vi "Tran to CRC.vi"(5 "CheckSum？":bool, 7 "Count":bool, 8 "MessageFrame":refnum<k21>="ESP_1\nLRA110", 9 "校验算法名称":string="Anti_Add", 11 "CAN_commd":dbl[](array[numeric])=[50.0, 1.0, 11.0, 0.0, 0.0, 0.0, 0.0, 0.0, 0.0] caption="data") -> (1 "Output CAN Command":u8[](array[numeric]) format="%x", 2 "校验值":u64 format="%.0x", 3 "SignalsArryOut":dbl[](array[numeric]))   [LabVIEW 2020]
panel:
  out "CAN_Command_U8":u8[](array[numeric]) format="%.0x"
  # "speedStatus"
  # "counter"
  # "speed"
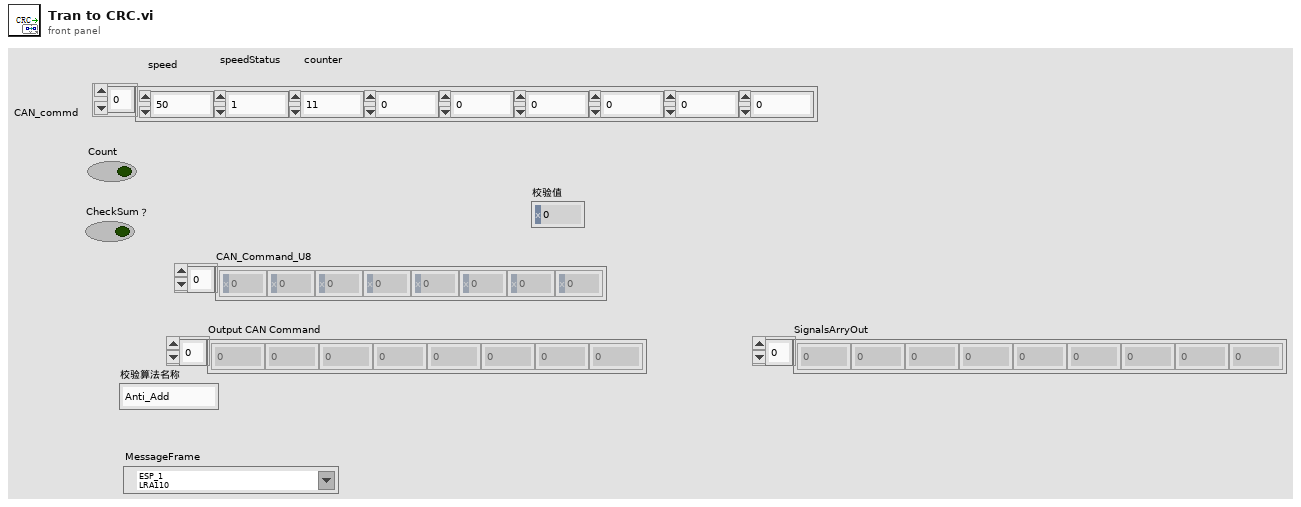
[diagram p1: front panel]
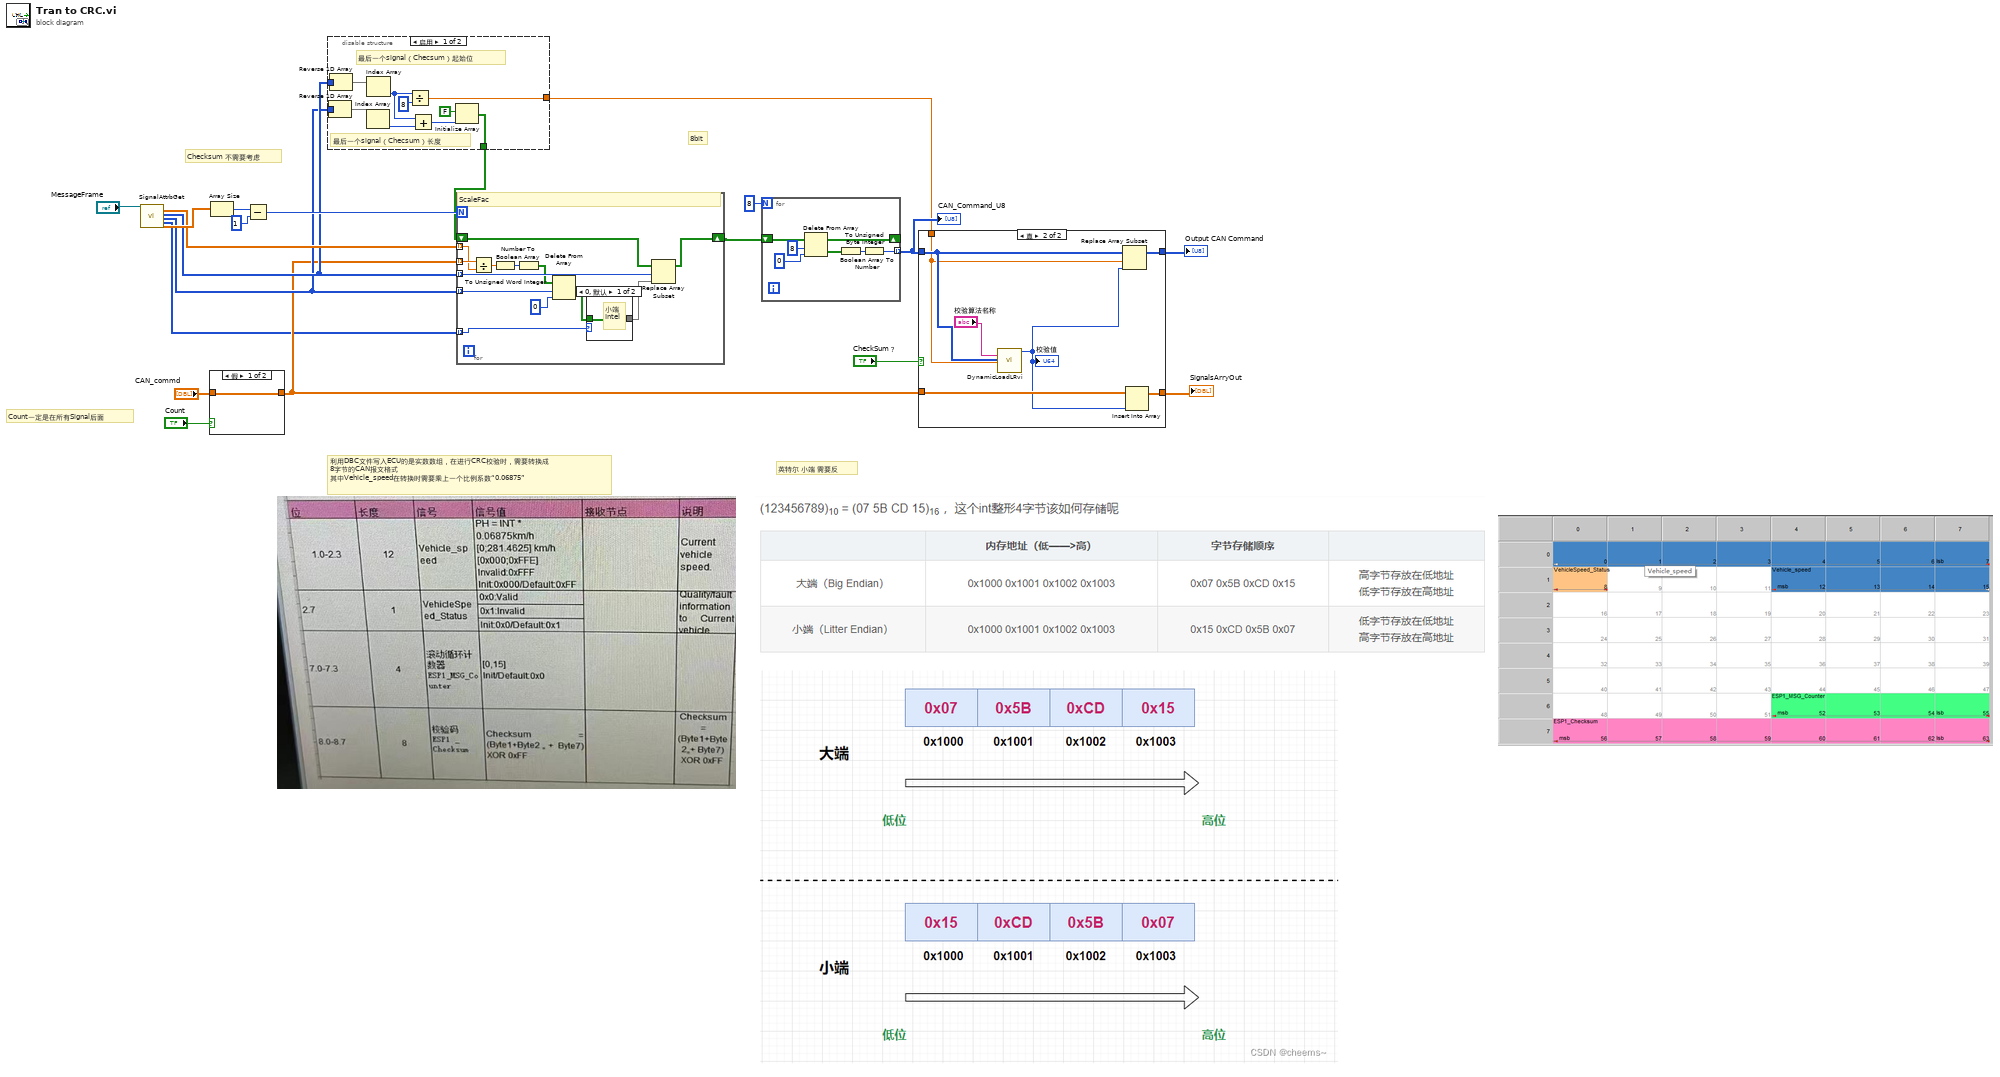
[diagram p0: block diagram]
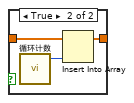
[diagram p3: hidden frame]
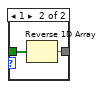
[diagram p5: hidden frame]
diagram:
  # "Count一定是在所有Signal后面"
  # "8bit"
  # "Checksum 不需要考虑"
  # "英特尔 小端 需要反"
  # "利用DBC文件写入ECU的是实数数组，在进行CRC校验时，需要转换成\n8字节的CAN报文格式\n其中Vehicle_speed在转换时需要乘上一个比例系数“0.06875”"
  n1 = call "SignalAttrbGet.vi"("MessageFrame"="MessageFrame") -> ("ScaleFac"=w15:dbl[], "StartBitArry"=w11:u32[], "Length"=w10:u32[], "DataType"=w1:u32[], "DefaultValue"=w18:dbl[])  [unwired: 13 in, 1 out]
  n2 = case shown="假" "Count" {
    tunnel: "CAN_commd" -> [w21 w24]
    tunnel: [w21 w22] -> w3
    frame False {
    }
    frame True {
      n3 = call "循环计数.vi"() -> ("循环计数"=w23:u8)  [unwired: 11 in]
      n4 = Insert Into Array(array=w24, new element=w23) -> (w22:dbl[])  [unwired: 1 in]
    }
  }
  n5 = Array Size(array=w18) -> (size(s)=w17:i32)
  n6 = Subtract(x=w17, y=1 ("x")) -> (x-y=w16:i32)
  n7 = disable-structure shown="启用" {
    disable-tunnel: w11 -> [w35 _]
    disable-tunnel: w10 -> [w34 _]
    disable-tunnel: [w30 _] -> w8
    disable-tunnel: [w25 _] -> w7
    frame Enabled {
      # "最后一个signal（Checsum）长度"
      # "最后一个signal（Checsum）起始位"
      n8 = Reverse 1D Array(array=w34) -> (reversed array=w32:u32[])
      n9 = Reverse 1D Array(array=w35) -> (reversed array=w33:u32[])
      n10 = Index Array(array=w32) -> (element=w28:u32)  [unwired: 1 in]
      n11 = Index Array(array=w33) -> (element=w29:u32)  [unwired: 1 in]
      n12 = Divide(x=w29, y=8) -> (x/y=w30:dbl)
      n13 = Add(x=w29, y=w28) -> (x+y=w26:u32)
      n14 = Initialize Array(FALSE, w26) -> (w25:bool[])
    }
    frame Disabled {
    }
  }
  n15 = for {
    N: w16 -> [_]
    tunnel: w3 -> [w48] mode=indexing
    tunnel: w15 -> [w47] mode=indexing
    tunnel: w11 -> [w42] mode=indexing
    shift-right: [w43] -> w12
    shift-left: w7 -> [w44]
    tunnel: w10 -> [w39] mode=indexing
    tunnel: w1 -> [w38] mode=indexing
    # "ScaleFac"
    n16 = Divide(x=w48, y=w47) -> (x/y=w46:dbl)
    n17 = To Unsigned Word Integer(number=w46) -> (unsigned 16bit integer=w45:u16)
    n18 = Number To Boolean Array(number=w45) -> (Boolean array=w40:bool[])
    n19 = Delete From Array(array=w40, length=w39, index=0) -> (deleted portion=w37:bool[])  [unwired: 1 out]
    n20 = case shown="0, 默认" w38 {
      tunnel: w37 -> [w49 w51]
      tunnel: [w49 w50] -> w36
      frame 0, Default {
        # "小端\nIntel"
      }
      frame 1 {
        n21 = Reverse 1D Array(array=w51) -> (reversed array=w50:bool[])
      }
    }
    n22 = Replace Array Subset(array=w44, new element=w36, index=w42) -> (w43:bool[])
  }
  n23 = for {
    N: 8 -> [_]
    shift-right: [w54] -> _
    shift-left: w12 -> [w58]
    tunnel: [w52] -> w9 mode=indexing
    n24 = Delete From Array(array=w58, length=8, index=0) -> (deleted portion=w55:bool[], array with subset deleted=w54:bool[])
    n25 = Boolean Array To Number(Boolean array=w55) -> (number=w53:u16)
    n26 = To Unsigned Byte Integer(number=w53) -> (unsigned 8bit integer=w52:u8)
  }
  "CAN_Command_U8" <- w9
  n27 = case shown="真" "CheckSum？" {
    tunnel: [w59 w67] -> w20
    tunnel: w9 -> [w59 w63]
    tunnel: w8 -> [_ w62]
    tunnel: w3 -> [w60 w66]
    tunnel: [w60 w65] -> w2
    frame False {
    }
    frame True {
      n28 = call "DynamicLoadLRvi.vi"("校验算法名称"="校验算法名称", "校验数据"=w63, "校验长度"=w62) -> ("校验值"=w61:u64)  [unwired: 16 in]
      "校验值" <- w61
      n29 = Replace Array Subset(array=w63, new element=w61, index=w62) -> (w67:u8[])
      n30 = Insert Into Array(array=w66, new element=w61) -> (w65:dbl[])  [unwired: 1 in]
    }
  }
  "Output CAN Command" <- w20
  "SignalsArryOut" <- w2
